vi "NIVS.FilterChannels.vi"(8 "error in (no error)":errorcluster, 11 "Cluster in":T1) -> (0 "error out":errorcluster, 3 "Cluster out":T1)   [LabVIEW 2015]
uses:
  Types/Main.StateVariables.ctl
  <vilib>/Utility/miscctls.llb/LVPositionTypeDef.ctl
  Types/Execute.UserEventRefs.ctl
  <vilib>/NI Veristand/Execution/Workspace/SystemStateRegEventRef.ctl
  <vilib>/NI Veristand/Execution/Workspace/Target State Info.ctl
  <vilib>/NI Veristand/Execution/Workspace/Target State.ctl
  <vilib>/NI Veristand/Execution/WaveformStreaming/Waveform Data Watcher Event Data (DBL).ctl
  <vilib>/NI Veristand/Execution/WaveformStreaming/WaveformStreamSpecification.ctl
  NationalInstruments.VeriStand.ClientAPI
  <vilib>/NI Veristand/Execution/Workspace/SystemStateEventRef.ctl
  <vilib>/NI Veristand/Execution/Workspace/WorkspaceAPI.ctl
  Types/UI.Object.ctl
  Types/Waveforms.Info.ctl
  <vilib>/NI Veristand/Execution/WaveformStreaming/Registered Waveform Streams Data Event Refnum (DBL).ctl
  <vilib>/NI Veristand/Execution/WaveformStreaming/WaveformDataWatcherDBL.ctl
  <vilib>/NI Veristand/Execution/WaveformStreaming/WaveformStreamingAPI.ctl
  NationalInstruments.VeriStand
  <vilib>/NI Veristand/Execution/Workspace/NI_VS Workspace ExecutionAPI.lvlib
  <vilib>/NI Veristand/Execution/WaveformStreaming/NI_VS Waveform Streaming Interface.lvlib
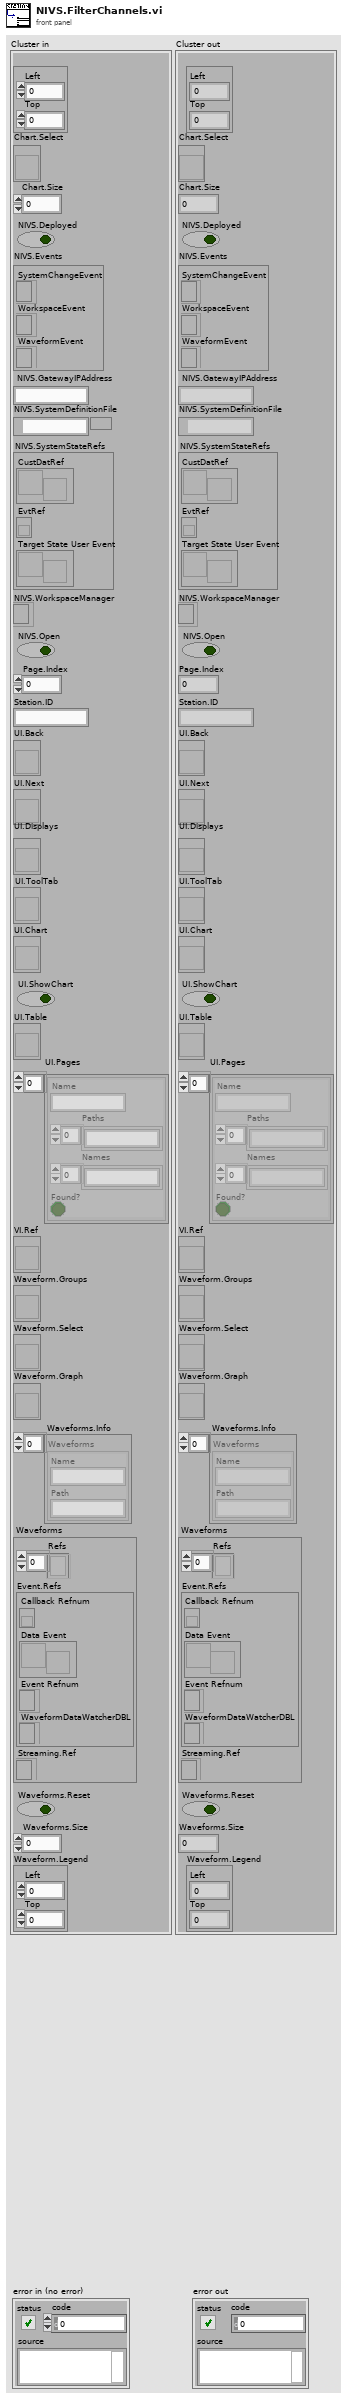
[diagram p1: front panel]
types:
  T1 = typedef "Main.StateVariables.ctl" = cluster{"Chart.Legend":T2, "Chart.Select":refnum<vi>, "Chart.Size":i32, "NIVS.Deployed":bool, "NIVS.Events":T3, "NIVS.GatewayIPAddress":string, "NIVS.SystemDefinitionFile":path, "NIVS.SystemStateRefs":T5, "NIVS.WorkspaceManager":T6, "NIVS.Open":bool, "Page.Index":u32, "Station.ID":string, "UI.Back":refnum<vi>, "UI.Next":refnum<vi>, "UI.Displays":refnum<vi>, "UI.ToolTab":refnum<vi>, "UI.Chart":refnum<vi>, "UI.ShowChart":bool, "UI.Table":refnum<vi>, "UI.Pages":T7[], "VI.Ref":refnum<vi>, "Waveform.Groups":refnum<vi>, "Waveform.Select":refnum<vi>, "Waveform.Graph":refnum<vi>, "Waveforms.Info":T8[], "Waveforms":cluster{"Refs":T9[], "Event.Refs":T10, "Streaming.Ref":T12}, "Waveforms.Reset":bool, "Waveforms.Size":i32, "Waveform.Legend":T2}
  T2 = typedef "LVPositionTypeDef.ctl" = cluster{"Left":i32, "Top":i32}
  T3 = typedef "Execute.UserEventRefs.ctl" = cluster{"SystemChangeEvent":T4, "WorkspaceEvent":refnum<event-registration>, "WaveformEvent":refnum<event-registration>}
  T4 = typedef "NI_VS Workspace ExecutionAPI.lvlib/SystemStateRegEventRef.ctl" = refnum<event-registration>
  T5 = typedef "NI_VS Workspace ExecutionAPI.lvlib/SystemStateEventRef.ctl" = cluster{"CustDatRef":refnum<user-event>, "EvtRef":refnum<k27>, "Target State User Event":refnum<user-event>}
  T6 = typedef "NI_VS Workspace ExecutionAPI.lvlib/WorkspaceAPI.ctl" = refnum<k24>
  T7 = typedef "UI.Object.ctl" = cluster{"Name":string, "Paths":string[], "Names":string[], "Found?":bool}
  T8 = typedef "Waveforms.Info.ctl" = cluster{"Name":string, "Path":string}
  T9 = typedef "NI_VS Waveform Streaming Interface.lvlib/WaveformStreamSpecification.ctl" = refnum<k24>
  T10 = typedef "NI_VS Waveform Streaming Interface.lvlib/Registered Waveform Streams Data Event Refnum (DBL).ctl" = cluster{"Callback Refnum":refnum<k27>, "Data Event":refnum<user-event>, "Event Refnum":refnum<event-registration>, "WaveformDataWatcherDBL":T11}
  T11 = typedef "NI_VS Waveform Streaming Interface.lvlib/WaveformDataWatcherDBL.ctl" = refnum<k24>
  T12 = typedef "NI_VS Waveform Streaming Interface.lvlib/WaveformStreamingAPI.ctl" = refnum<k24>
  T13 = typedef "NI_VS Workspace ExecutionAPI.lvlib/NodeInfo.ctl" = cluster{"Name":string, "FullPath":string, "Type":string, "IsChannel":bool, "Channel":cluster{"Unit":string, "Readable":bool, "Writable":bool, "Faultable":bool, "Scalable":bool, "RowDim":u32, "ColumnDim":u32, "Value Table Names":string[], "Value Table Values":dbl[]}, "IsWaveform":bool, "Waveform":cluster{"DataType":T14}}
  T14 = typedef "NI_VS Workspace ExecutionAPI.lvlib/Waveform Data Type.ctl" = enum16{"Double", "ComplexDouble"}
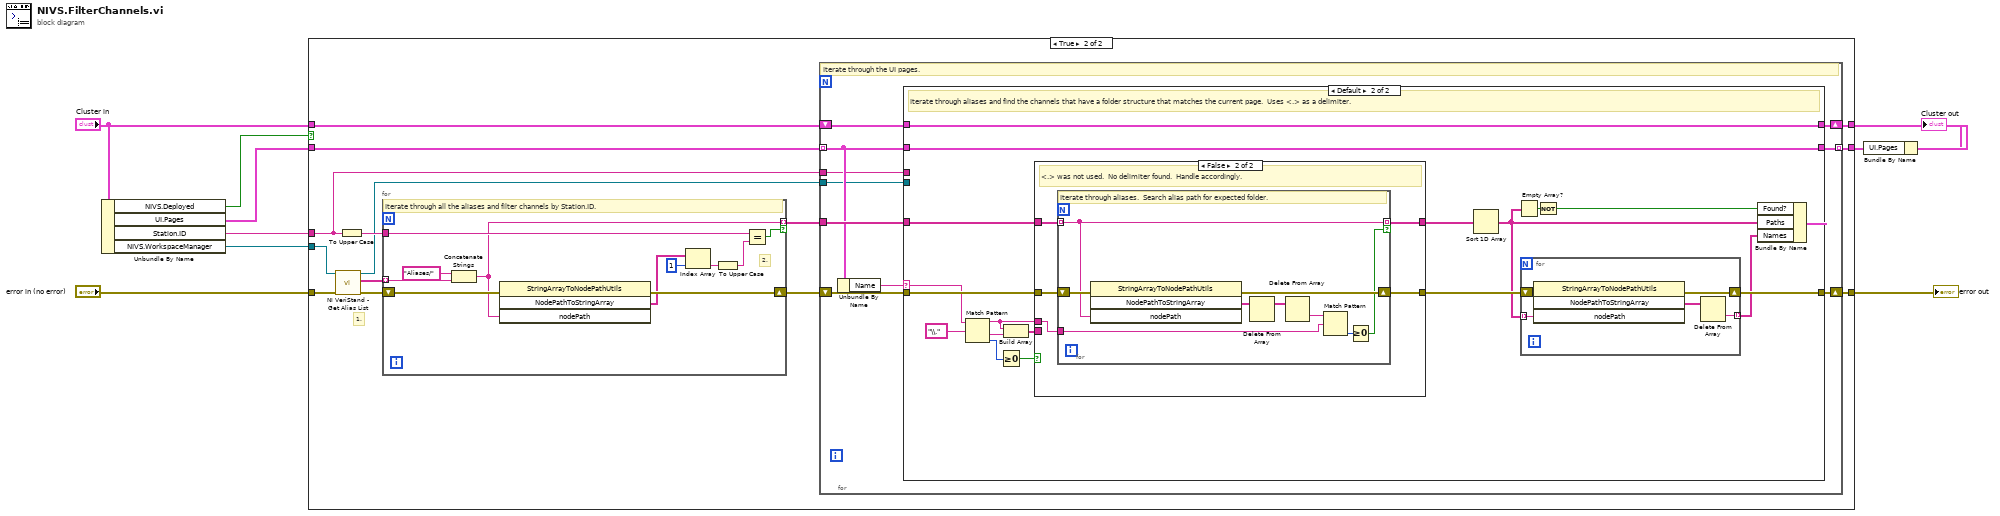
[diagram p0: block diagram]
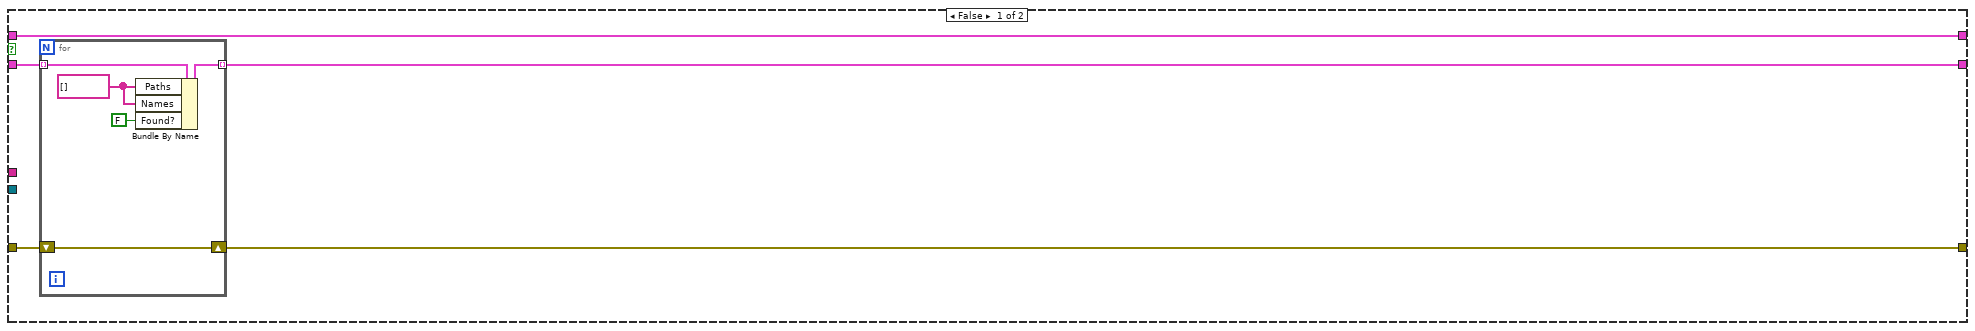
[diagram p2: hidden frame]
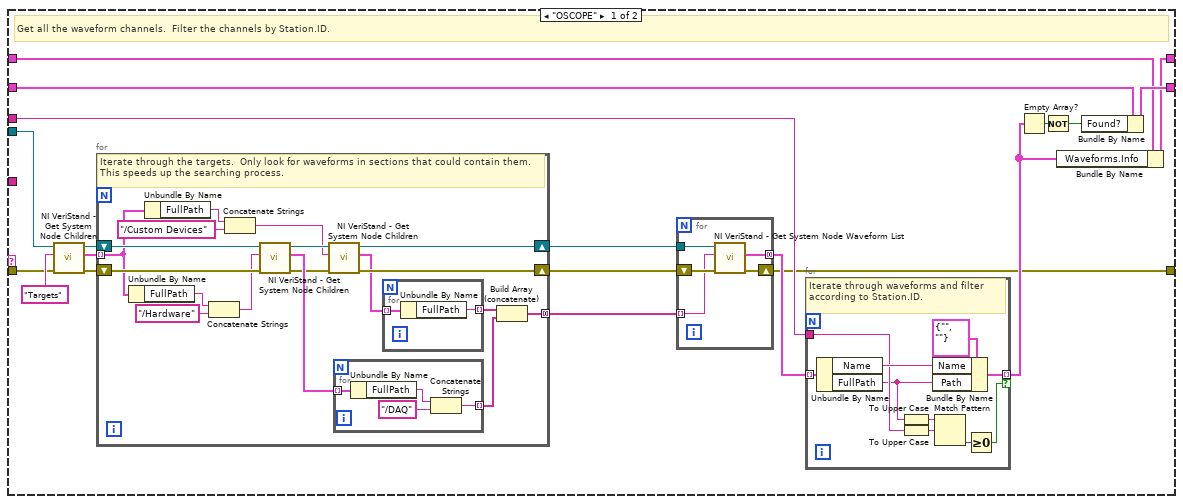
[diagram p3: hidden frame]
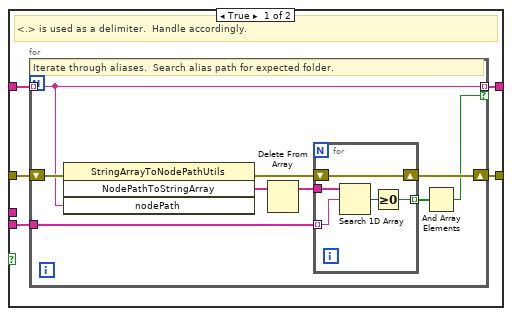
[diagram p4: hidden frame]
diagram:
  n1 = Unbundle By Name("Cluster in") -> ("NIVS.Deployed"=w6:bool, "UI.Pages"=w5:T7[], "Station.ID"=w8:string, "NIVS.WorkspaceManager"=w9:T6)
  n2 = case shown="True" w6 {
    tunnel: "error in (no error)" -> [w13 w34]
    tunnel: w9 -> [_ w33]
    tunnel: w8 -> [_ w23]
    tunnel: w5 -> [w15 w28]
    tunnel: [w12 w26] -> w7
    tunnel: [w14 w25] -> w4
    tunnel: "Cluster in" -> [w11 w22]
    tunnel: [w11 w21] -> w1
    frame False {
      n3 = for {
        shift-right: [w17] -> w12
        shift-left: w13 -> [w17]
        tunnel: w15 -> [w19] mode=indexing
        tunnel: [w18] -> w14 mode=indexing
        w20 = string[] [] ("Channels")
        n4 = Bundle By Name(cluster=w19, "Paths"=w20, "Names"=w20, "Found?"=FALSE) -> (w18:T7)
      }
    }
    frame True {
      # "1."
      n5 = call <vilib>:"NI VeriStand - Get Alias List.vi"("error in (no error)"=w34, "WorkspaceManager in"=w33) -> ("error out"=w31:errorcluster, "Aliases"=w32:string[], "WorkspaceManager out"=w24:T6)  [unwired: 6 in, 1 out]
      n6 = To Upper Case(1:w23) -> (0:w30:string)
      n7 = for {
        tunnel: w32 -> [w37] mode=indexing
        shift-right: [w39] -> w27
        shift-left: w31 -> [w45]
        tunnel: w30 -> [w41]
        tunnel: [w36] -> w29 mode=indexing if=w40
        # "2."
        # "Iterate through all the aliases and filter channels by Station.ID."
        n8 = Concatenate Strings("Aliases/", w37) -> (w36:string)
        n9 = invoke class="StringArrayToNodePathUtils" method="NodePathToStringArray"(error in=w45, "nodePath"=w36) -> (error out=w39:errorcluster, "NodePathToStringArray"=w38:string[])  [unwired: 2 in, 2 out]
        n10 = Index Array(array=w38, index=1) -> (element=w43:string)
        n11 = To Upper Case(1:w43) -> (0:w42:string)
        n12 = Equal?(x=w41, y=w42) -> (x = y?=w40:bool)
      }
      n13 = for {
        tunnel: w29 -> [w55]
        shift-right: [w52] -> w26
        shift-left: w27 -> [w53]
        tunnel: w28 -> [w54] mode=indexing
        tunnel: [w51] -> w25 mode=indexing
        tunnel: w24 -> [w49]
        tunnel: w23 -> [w48]
        shift-right: [w46] -> w21
        shift-left: w22 -> [w47]
        # "Iterate through the UI pages."
        n14 = Unbundle By Name(w54) -> ("Name"=w50:string)
        n15 = case shown="Default" w50 {
          selector: w50 -> [_ w118]
          tunnel: w55 -> [_ w132]
          tunnel: w54 -> [w74 w131]
          tunnel: w53 -> [w57 w130]
          tunnel: [w58 w129] -> w52
          tunnel: [w73 w128] -> w51
          tunnel: w49 -> [w56 _]
          tunnel: w48 -> [w72 _]
          tunnel: w47 -> [w71 w114]
          tunnel: [w70 w114] -> w46
          frame "OSCOPE" {
            # "Get all the waveform channels.  Filter the channels by Station.ID."
            n16 = call <vilib>:"NI VeriStand - Get System Node Children.vi"("error in (no error)"=w57, "Node"="Targets", "WorkspaceManager in"=w56) -> ("error out"=w64:errorcluster, "Nodes"=w65:T13[], "WorkspaceManager out"=w63:T6)  [unwired: 6 in]
            n17 = for {
              tunnel: w65 -> [w85] mode=indexing
              shift-right: [w89] -> w62
              shift-left: w64 -> [w95]
              shift-right: [w88] -> w61
              shift-left: w63 -> [w94]
              tunnel: [w81] -> w60 mode=concatenating
              # "Iterate through the targets.  Only look for waveforms in sections that could contain them.  This speeds up the searching process."
              n18 = Unbundle By Name(w85) -> ("FullPath"=w97:string)
              n19 = Unbundle By Name(w85) -> ("FullPath"=w86:string)
              n20 = Concatenate Strings(w97, "/Hardware" ("string")) -> (w93:string)
              n21 = Concatenate Strings(w86, "/Custom Devices" ("string")) -> (w84:string)
              n22 = call <vilib>:"NI VeriStand - Get System Node Children.vi"("error in (no error)"=w95, "Node"=w93, "WorkspaceManager in"=w94) -> ("error out"=w90:errorcluster, "Nodes"=w92:T13[], "WorkspaceManager out"=w91:T6)  [unwired: 6 in]
              n23 = call <vilib>:"NI VeriStand - Get System Node Children.vi"("error in (no error)"=w90, "Node"=w84, "WorkspaceManager in"=w91) -> ("error out"=w89:errorcluster, "Nodes"=w83:T13[], "WorkspaceManager out"=w88:T6)  [unwired: 6 in]
              n24 = for {
                tunnel: w92 -> [w103] mode=indexing
                tunnel: [w100] -> w80 mode=indexing
                n25 = Unbundle By Name(w103) -> ("FullPath"=w101:string)
                n26 = Concatenate Strings(w101, "/DAQ" ("string")) -> (w100:string)
              }
              n27 = for {
                tunnel: w83 -> [w99] mode=indexing
                tunnel: [w98] -> w82 mode=indexing
                n28 = Unbundle By Name(w99) -> ("FullPath"=w98:string)
              }
              n29 = Build Array (concatenate)(w82, w80) -> (w81:string[])
            }
            n30 = for {
              tunnel: w61 -> [w79]
              tunnel: w60 -> [w77] mode=indexing
              shift-right: [w76] -> w58
              shift-left: w62 -> [w78]
              tunnel: [w75] -> w59 mode=concatenating
              n31 = call <vilib>:"NI VeriStand - Get System Node Waveform List.vi"("error in (no error)"=w78, "StartNode (\"\")"=w77, "WorkspaceManager in"=w79) -> ("error out"=w76:errorcluster, "Waveforms"=w75:T13[])  [unwired: 6 in, 1 out]
            }
            n32 = for {
              tunnel: w59 -> [w113] mode=indexing
              tunnel: [w111] -> w68 mode=indexing if=w108
              tunnel: w72 -> [w107]
              # "Iterate through waveforms and filter according to Station.ID."
              n33 = Unbundle By Name(w113) -> ("Name"=w112:string, "FullPath"=w105:string)
              n34 = To Upper Case(1:w105) -> (0:w104:string)
              n35 = To Upper Case(1:w107) -> (0:w106:string)
              n36 = Bundle By Name(cluster=T8 {"Name"="", "Path"=""} ("Waveforms"), "Name"=w112, "Path"=w105) -> (w111:T8)
              n37 = Match Pattern(string=w104, regular expression=w106) -> (offset past match=w109:i32)  [unwired: 1 in, 3 out]
              n38 = Greater Or Equal To 0?(x=w109) -> (x >= 0?=w108:bool)
            }
            n39 = Empty Array?(array=w68) -> (empty?=w69:bool)
            n40 = Not(x=w69) -> (.not. x?=w67:bool)
            n41 = Bundle By Name(cluster=w71, "Waveforms.Info"=w68) -> (w70:T1)
            n42 = Bundle By Name(cluster=w74, "Found?"=w67) -> (w73:T7)
          }
          frame Default {
            # "Iterate through aliases and find the channels that have a folder structure that matches the current page.  Uses <.> as a delimiter."
            n43 = Match Pattern(string=w118, regular expression="\\.") -> (before substring=w121:string, after substring=w125:string, offset past match=w126:i32)  [unwired: 1 in, 1 out]
            n44 = Greater Or Equal To 0?(x=w126) -> (x >= 0?=w123:bool)
            n45 = Build Array(w121, w125) -> (w122:string[])
            n46 = case shown="False" w123 {
              tunnel: w132 -> [w137 w156]
              tunnel: w130 -> [w136 w155]
              tunnel: w122 -> [w135 _]
              tunnel: [w134 w154] -> w124
              tunnel: [w133 w153] -> w119
              tunnel: w121 -> [_ w152]
              frame True {
                # "<.> is used as a delimiter.  Handle accordingly."
                n47 = for {
                  tunnel: w137 -> [w141] mode=indexing
                  shift-right: [w142] -> w133
                  shift-left: w136 -> [w146]
                  tunnel: w135 -> [w145]
                  tunnel: [w141] -> w134 mode=indexing if=w140
                  # "Iterate through aliases.  Search alias path for expected folder."
                  n48 = invoke class="StringArrayToNodePathUtils" method="NodePathToStringArray"(error in=w146, "nodePath"=w141) -> (error out=w144:errorcluster, "NodePathToStringArray"=w139:string[])  [unwired: 2 in, 2 out]
                  n49 = Delete From Array(array=w139) -> (array with subset deleted=w138:string[])  [unwired: 2 in, 1 out]
                  n50 = for {
                    tunnel: w138 -> [w151]
                    tunnel: w145 -> [w150] mode=indexing
                    shift-right: [w148] -> w142
                    shift-left: w144 -> [w148]
                    tunnel: [w147] -> w143 mode=indexing
                    n51 = Search 1D Array(1D array=w151, element=w150) -> (index of element=w149:i32)  [unwired: 1 in]
                    n52 = Greater Or Equal To 0?(x=w149) -> (x >= 0?=w147:bool)
                  }
                  n53 = And Array Elements(Boolean array=w143) -> (logical AND=w140:bool)
                }
              }
              frame False {
                # "<.> was not used.  No delimiter found.  Handle accordingly."
                n54 = for {
                  tunnel: w156 -> [w161] mode=indexing
                  shift-right: [w162] -> w153
                  shift-left: w155 -> [w165]
                  tunnel: w152 -> [w163]
                  tunnel: [w161] -> w154 mode=indexing if=w159
                  # "Iterate through aliases.  Search alias path for expected folder."
                  n55 = invoke class="StringArrayToNodePathUtils" method="NodePathToStringArray"(error in=w165, "nodePath"=w161) -> (error out=w162:errorcluster, "NodePathToStringArray"=w164:string[])  [unwired: 2 in, 2 out]
                  n56 = Delete From Array(array=w164) -> (array with subset deleted=w158:string[])  [unwired: 2 in, 1 out]
                  n57 = Delete From Array(array=w158) -> (deleted portion=w157:string)  [unwired: 2 in, 1 out]
                  n58 = Match Pattern(string=w157, regular expression=w163) -> (offset past match=w160:i32)  [unwired: 1 in, 3 out]
                  n59 = Greater Or Equal To 0?(x=w160) -> (x >= 0?=w159:bool)
                }
              }
            }
            n60 = Sort 1D Array(array=w124) -> (sorted array=w117:string[])
            n61 = Empty Array?(array=w117) -> (empty?=w116:bool)
            n62 = for {
              tunnel: [w169] -> w120 mode=indexing
              shift-right: [w167] -> w129
              shift-left: w119 -> [w168]
              tunnel: w117 -> [w166] mode=indexing
              n63 = invoke class="StringArrayToNodePathUtils" method="NodePathToStringArray"(error in=w168, "nodePath"=w166) -> (error out=w167:errorcluster, "NodePathToStringArray"=w170:string[])  [unwired: 2 in, 2 out]
              n64 = Delete From Array(array=w170) -> (deleted portion=w169:string)  [unwired: 2 in, 1 out]
            }
            n65 = Not(x=w116) -> (.not. x?=w115:bool)
            n66 = Bundle By Name(cluster=w131, "Found?"=w115, "Paths"=w117, "Names"=w120) -> (w128:T7)
          }
        }
      }
    }
  }
  "error out" <- w7
  n67 = Bundle By Name(cluster=w1, "UI.Pages"=w4) -> (→"Cluster out":T1)
